vi "Supported-actions.vi"(8 "error in (no error)":errorcluster, 10 "Supported action?":T1=enum."Move - Relative", 11 "Motor in":refnum<class "Motor-Zaxis.lvclass">) -> (0 "error out":errorcluster, 1 "Supported?":bool, 2 "Supported actions":T1[](array[typedef]), 3 "Motor out":refnum<class "Motor-Zaxis.lvclass">)   [LabVIEW 2013, in "PowderDeposition.lvlib" / "Motor-Zaxis.lvclass"]
uses:
  Motor-Zaxis.lvclass
  Action/Motor-actions.ctl
  Action/Action.lvclass
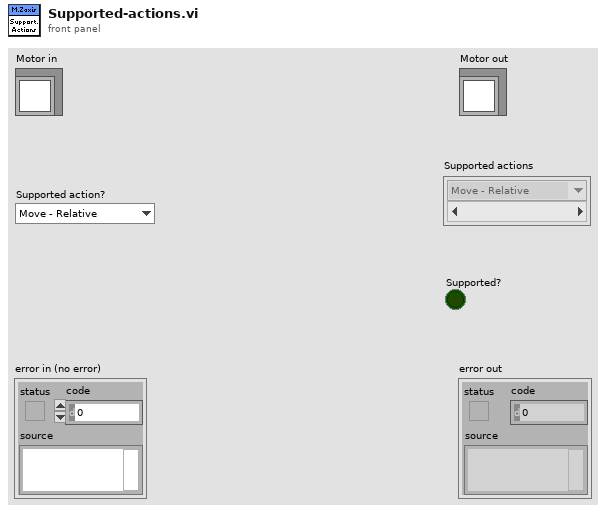
[diagram p1: front panel]
types:
  T1 = typedef "PowderDeposition.lvlib/Action.lvclass/Motor-actions.ctl" = enum16{"Move - Absolute", "Move - Relative", "Move - Timer", "Wait", "Home", "Substrate", "Sieve", "Stop"}
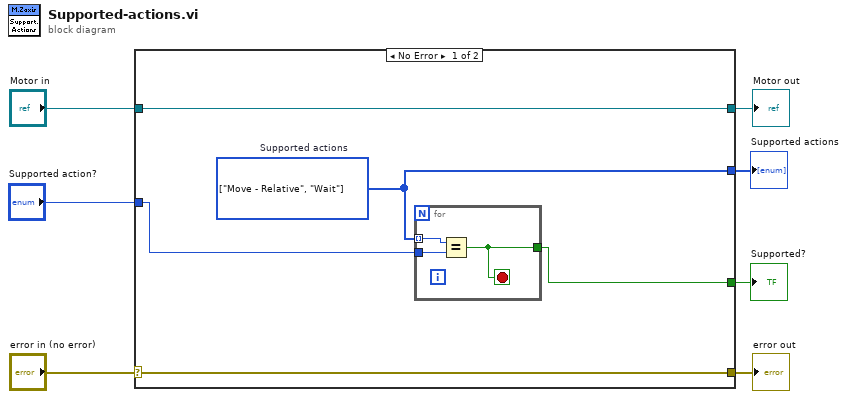
[diagram p0: block diagram]
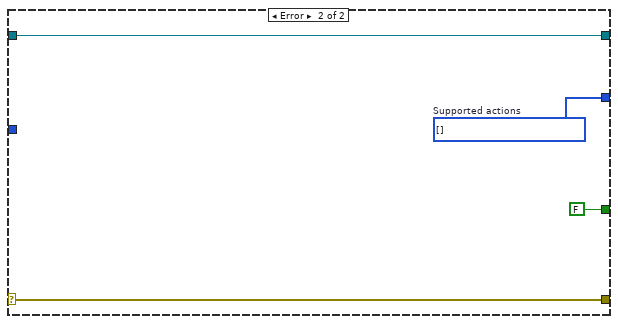
[diagram p2: hidden frame]
diagram:
  n1 = case shown="No Error" "error in (no error)" {
    selector: "error in (no error)" -> [w11 w19]
    tunnel: [w11 w19] -> w6
    tunnel: [w12 w18] -> w4
    tunnel: "Motor in" -> [w12 w18]
    tunnel: "Supported action?" -> [w9 _]
    tunnel: [w10 w17] -> w2
    tunnel: [w8 FALSE] -> w1
    frame No Error {
      w10 = T1[] [enum."Move - Relative", enum."Wait"] items=["Move - Absolute", "Move - Relative", "Move - Timer", "Wait", "Home", "Substrate", "Sieve", "Stop"]  # Supported actions
      n2 = for {
        tunnel: w10 -> [w15] mode=indexing
        tunnel: w9 -> [w14]
        tunnel: [w13] -> w8
        stop <- w13 stop-if-true
        n3 = Equal?(x=w15, y=w14) -> (x = y?=w13:bool)
      }
    }
    frame Error {
      w17 = T1[] [] items=["Move - Absolute", "Move - Relative", "Move - Timer", "Wait", "Home", "Substrate", "Sieve", "Stop"]  # Supported actions
    }
  }
  "error out" <- w6
  "Motor out" <- w4
  "Supported actions" <- w2
  "Supported?" <- w1
